vi "SSP - get control details.vi"(8 "error in (no error)":errorcluster, 11 "JSON string":string) -> (0 "error out":errorcluster, 3 "value":string)   [LabVIEW 2020, in "ui-testing.lvlib"]
doc: "copyright: Thomas Zilliox©"
uses:
  ui-testing.lvlib
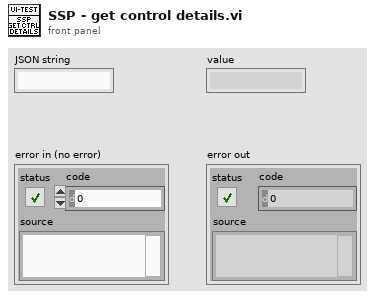
[diagram p1: front panel]
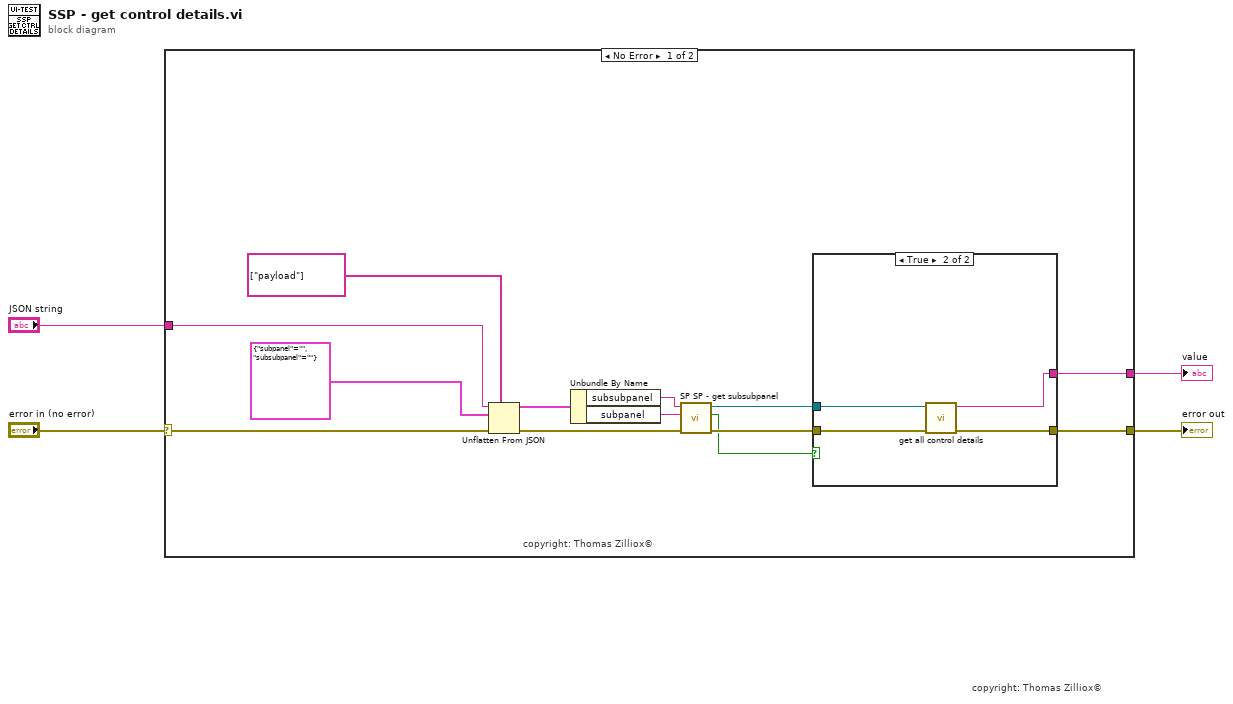
[diagram p0: block diagram]
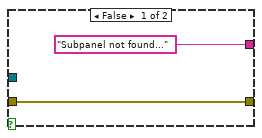
[diagram p2: hidden frame]
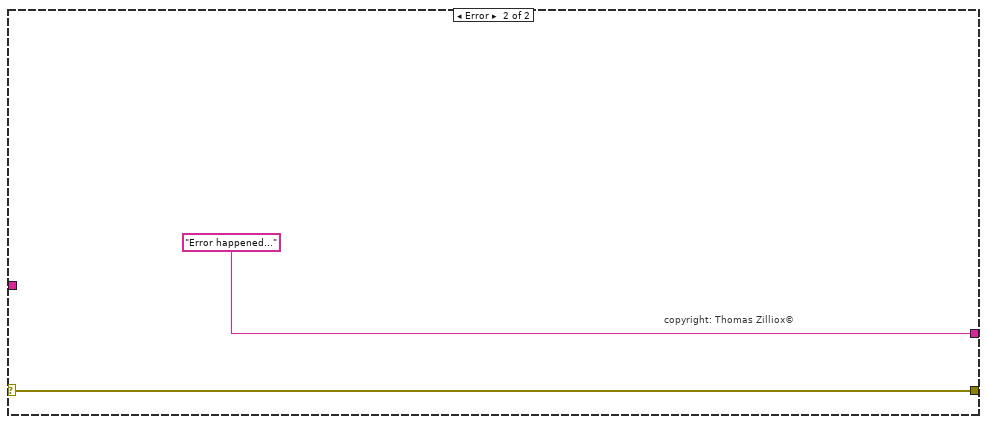
[diagram p3: hidden frame]
diagram:
  # "copyright: Thomas Zilliox©"
  n1 = case shown="No Error" "error in (no error)" {
    selector: "error in (no error)" -> [w12 w25]
    tunnel: "JSON string" -> [w13 _]
    tunnel: [w17 w25] -> w3
    tunnel: [w16 "Error happened..."] -> w1
    frame No Error {
      # "copyright: Thomas Zilliox©"
      n2 = Unflatten From JSON(path=string[] ["payload"], JSON string=w13, type and defaults=cluster{"subpanel":string, "subsubpanel":string} {"subpanel"="", "subsubpanel"=""}, error in (no error)=w12) -> (value=w11:cluster{"subpanel":string, "subsubpanel":string}, error out=w8:errorcluster)  [unwired: 3 in]
      n3 = Unbundle By Name(w11) -> ("subsubpanel"=w10:string, "subpanel"=w9:string)
      n4 = call "SP SP - get subsubpanel.vi"("error in (no error)"=w8, "subpanel"=w9, "subsubpanel"=w10) -> ("error out"=w7:errorcluster, "SubSubPanel found"=w5:bool, "SubSubPanel VI"=w6:refnum<vi>)  [unwired: 5 in, 1 out]
      n5 = case shown="True" w5 {
        tunnel: w7 -> [w18 w22]
        tunnel: [w18 w21] -> w17
        tunnel: ["Subpanel not found..." ("Name") w20] -> w16
        tunnel: w6 -> [_ w23]
        frame False {
        }
        frame True {
          n6 = call "get all control details.vi"("error in"=w22, "VI (Caller)"=w23) -> ("error out"=w21:errorcluster, "Control details"=w20:string)  [unwired: 8 in]
        }
      }
    }
    frame Error {
      # "copyright: Thomas Zilliox©"
    }
  }
  "error out" <- w3
  "value" <- w1
